vi "Load FPGA Interface.vi"(8 "error in (no error)":errorcluster, 11 "Guardian in":refnum<class "Guardian.lvclass">) -> (0 "error out":errorcluster, 3 "Guardian out":refnum<class "Guardian.lvclass">)   [LabVIEW 2026, in "TALOS.lvlib" / "Guardian.lvlib" / "Guardian.lvclass"]
uses:
  Guardian.lvclass
  d88df795-0ef9-4a38-95d7-8ccd969dbc7e.vi
  58b126a1-d1b0-4ff9-95ea-5941d609dff4.vi
  58b126a1-d1b0-4ff9-95ea-5941d609dff4.vi/d4db2432-cc9c-482c-8957-dac855435ef6.vi
  58b126a1-d1b0-4ff9-95ea-5941d609dff4.vi/86fbf154-bd7b-49a2-8ab2-a837b2a95f24.vi
  58b126a1-d1b0-4ff9-95ea-5941d609dff4.vi/3b95b01e-1ec2-4565-bcd9-7606a5281010.vi
  58b126a1-d1b0-4ff9-95ea-5941d609dff4.vi/96a08935-737a-44b2-979c-a81d56408f7e.vi
  58b126a1-d1b0-4ff9-95ea-5941d609dff4.vi/d4db2432-cc9c-482c-8957-dac855435ef6.vi/6eaecd13-6e48-4772-a921-b51ebdf84d88.vi
  58b126a1-d1b0-4ff9-95ea-5941d609dff4.vi/d4db2432-cc9c-482c-8957-dac855435ef6.vi/d2d5f2b7-06f4-47f6-971c-049c3fdbb653.vi
  58b126a1-d1b0-4ff9-95ea-5941d609dff4.vi/3b95b01e-1ec2-4565-bcd9-7606a5281010.vi/6eaecd13-6e48-4772-a921-b51ebdf84d88.vi
  58b126a1-d1b0-4ff9-95ea-5941d609dff4.vi/3b95b01e-1ec2-4565-bcd9-7606a5281010.vi/d2d5f2b7-06f4-47f6-971c-049c3fdbb653.vi
  58b126a1-d1b0-4ff9-95ea-5941d609dff4.vi/96a08935-737a-44b2-979c-a81d56408f7e.vi/6eaecd13-6e48-4772-a921-b51ebdf84d88.vi
  58b126a1-d1b0-4ff9-95ea-5941d609dff4.vi/96a08935-737a-44b2-979c-a81d56408f7e.vi/d2d5f2b7-06f4-47f6-971c-049c3fdbb653.vi
  <vilib>/Comparison/Less/Less Functor/Less Functor.lvclass
  TALOS.lvlib
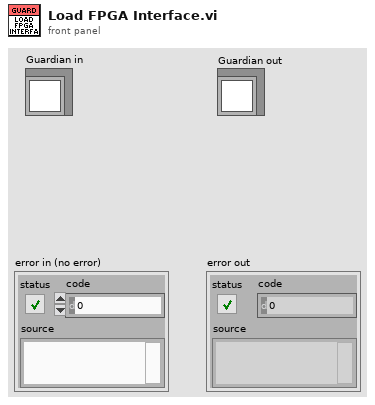
[diagram p1: front panel]
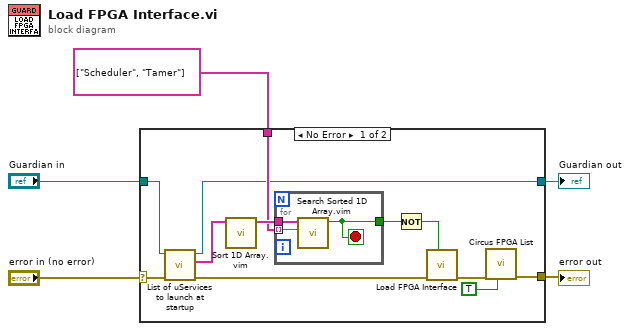
[diagram p0: block diagram]
diagram:
  n1 = case shown="No Error" "error in (no error)" {
    selector: "error in (no error)" -> [w14 w22]
    tunnel: [w16 w22] -> w5
    tunnel: "Guardian in" -> [w13 w21]
    tunnel: [w8 w21] -> w2
    tunnel: string[] ["Scheduler", "Tamer"] -> [w10 _]
    frame No Error {
      n2 = call "List of uServices to launch at startup.vi"("error in (no error)"=w14, "Guardian in"=w13) -> ("error out"=w9:errorcluster, "Array"=w12:string[], "Guardian out"=w8:refnum<class "Guardian.lvclass">)  [unwired: 7 in]
      n3 = call "Sort 1D Array.vim"("unsorted array"=w12) -> ("sorted array"=w11:string[])  [unwired: 10 in]
      n4 = for {
        tunnel: w11 -> [w20]
        tunnel: w10 -> [w19] mode=indexing
        tunnel: [w18] -> w7
        stop <- w18 stop-if-true
        n5 = call "Search Sorted 1D Array.vim"("element"=w19, "sorted 1D array"=w20) -> ("found?"=w18:bool)  [unwired: 8 in, 1 out]
      }
      n6 = Not(x=w7) -> (.not. x?=w6:bool)
      n7 = call "Load FPGA Interface.vi"("Don't load"=w6, "error in (no error)"=w9) -> ("error out"=w15:errorcluster)  [unwired: 9 in]
      n8 = call "Circus FPGA List.vi"("Init"=TRUE, "error in (no error)"=w15) -> ("error out"=w16:errorcluster)  [unwired: 8 in, 1 out]
    }
    frame Error {
    }
  }
  "error out" <- w5
  "Guardian out" <- w2
